vi "Read Attributes.vi"(11 "Return Device Generation Mode Msg":refnum<class "Return Device Generation Mode Msg.lvclass">) -> (2 "Payload":cluster{"DeviceID":u64, "Generation Mode":T1})   [LabVIEW 2016, in "Optimization Framework.lvlib" / "Return Device Generation Mode Msg.lvclass"]
uses:
  Return Device Generation Mode Msg.lvclass
  Optimization/Controls/Device Generation Mode.ctl
  Return Device Generation Mode Msg.lvclass/Return Device Generation Mode Msg.ctl
  Optimization/Optimization.lvclass
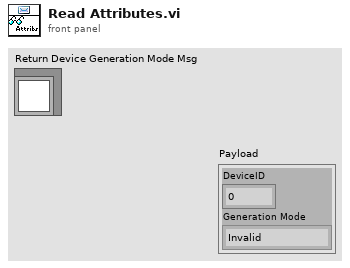
[diagram p1: front panel]
types:
  T1 = typedef "Optimization Framework.lvlib/Optimization.lvclass/Device Generation Mode.ctl" = enum16{"Invalid", "PQ", "Droop", "PV", "PF", "VF"}
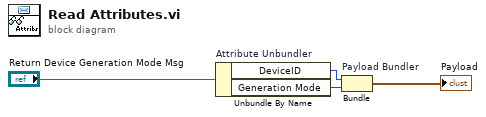
[diagram p0: block diagram]
diagram:
  n1 = Unbundle By Name "Attribute Unbundler"("Return Device Generation Mode Msg") -> ("DeviceID"=w2:u64, "Generation Mode"=w1:T1)
  n2 = Bundle "Payload Bundler"("DeviceID"=w2, "Generation Mode"=w1) -> (→"Payload":cluster{"DeviceID":u64, "Generation Mode":T1})  [unwired: 1 in]
